vi "nanocal -- nuclear schottky fit -- 2x2 -- V9.vi"() -> ()   [LabVIEW 2021] (continued)
\"στS\" -> 0.003636352111   ,  \"στN\" -> 0.036322417436    |>   , \n\"IDS0184_210310_RAW_cal__sam_\" ->   <|    \"ζ\" -> 0.215697702358   ,  \"τ1\" -> 0.095971807771   ,  \"τS\" -> 0.069319630290   ,  \"τN\" -> 0.366712218878   ,  \"τC\" -> 0.001526252261   ,  \"κ0\" -> 0.000000000784   ,  \"mm1\" -> 0.000266752031   ,  \"mm2\" -> 0.013373263674   ,  \"mm3\" -> 0.613940961515   ,  \"T\" -> 0.148000000000   ,  \"B\" -> 12.000000000000   ,  \"θ\" -> 90.000000000000   ,  \"Reoff\" -> 0.000000000000   ,  \"Imoff\" -> 0.000000000000   ,  \"στ1\" -> 0.000000000000   ,  \"στS\" -> 0.000000000000   ,  \"στN\" -> 0.000000000000    |>   , \n\"IDS0185_210310_RAW_cal__ref_\" ->   <|    \"ζ\" -> 0.175626342721   ,  \"τ1\" -> 0.068013297959   ,  \"τS\" -> 0.031455235747   ,  \"τN\" -> 0.088683010169   ,  \"τC\" -> 0.000955517601   ,  \"κ0\" -> 0.000000001059   ,  \"mm1\" -> 0.000139645447   ,  \"mm2\" -> 0.013049177780   ,  \"mm3\" -> 0.197017679000   ,  \"T\" -> 0.197000000000   ,  \"B\" -> 12.000000000000   ,  \"θ\" -> 90.000000000000   ,  \"Reoff\" -> -34453061.224489793200   ,  \"Imoff\" -> 0.000000000000   ,  \"στ1\" -> 0.004608846817   ,  \"στS\" -> 0.000610901813   ,  \"στN\" -> 0.004550742696    |>   , \n\"IDS0185_210310_RAW_cal__sam_\" ->   <|    \"ζ\" -> 0.139117463690   ,  \"τ1\" -> 0.070330410174   ,  \"τS\" -> 0.040829719954   ,  \"τN\" -> 0.122434321115   ,  \"τC\" -> 0.001436112939   ,  \"κ0\" -> 0.000000001208   ,  \"mm1\" -> 0.000170710071   ,  \"mm2\" -> 0.013785404893   ,  \"mm3\" -> 0.243787328523   ,  \"T\" -> 0.197000000000   ,  \"B\" -> 12.000000000000   ,  \"θ\" -> 90.000000000000   ,  \"Reoff\" -> 0.000000000000   ,  \"Imoff\" -> 0.000000000000   ,  \"στ1\" -> 0.000000000000   ,  \"στS\" -> 0.000000000000   ,  \"στN\" -> 0.000000000000    |>   , \n\"IDS0186_210310_RAW_cal__ref_\" ->   <|    \"ζ\" -> 0.101402144849   ,  \"τ1\" -> 0.051259228694   ,  \"τS\" -> 0.026993470844   ,  \"τN\" -> 0.035386078801   ,  \"τC\" -> 0.001239642629   ,  \"κ0\" -> 0.000000001363   ,  \"mm1\" -> 0.000109940153   ,  \"mm2\" -> 0.014897296966   ,  \"mm3\" -> 0.106196603977   ,  \"T\" -> 0.249000000000   ,  \"B\" -> 12.000000000000   ,  \"θ\" -> 90.000000000000   ,  \"Reoff\" -> -14000000.000000000000   ,  \"Imoff\" -> 0.000000000000   ,  \"στ1\" -> 0.003203070466   ,  \"στS\" -> 0.000314021587   ,  \"στN\" -> 0.001544007051    |>   , \n\"IDS0186_210310_RAW_cal__sam_\" ->   <|    \"ζ\" -> 0.079912790251   ,  \"τ1\" -> 0.053932962768   ,  \"τS\" -> 0.033847624645   ,  \"τN\" -> 0.047947649984   ,  \"τC\" -> 0.001828917906   ,  \"κ0\" -> 0.000000001546   ,  \"mm1\" -> 0.000129305669   ,  \"mm2\" -> 0.016142481427   ,  \"mm3\" -> 0.127821856832   ,  \"T\" -> 0.249000000000   ,  \"B\" -> 12.000000000000   ,  \"θ\" -> 90.000000000000   ,  \"Reoff\" -> 0.000000000000   ,  \"Imoff\" -> 0.000000000000   ,  \"στ1\" -> 0.000000000000   ,  \"στS\" -> 0.000000000000   ,  \"στN\" -> 0.000000000000    |>   , \n\"IDS0187_210310_RAW_cal__ref_\" ->   <|    \"ζ\" -> 0.070400852728   ,  \"τ1\" -> 0.043683571138   ,  \"τS\" -> 0.023747872987   ,  \"τN\" -> 0.017566907569   ,  \"τC\" -> 0.001811397979   ,  \"κ0\" -> 0.000000001742   ,  \"mm1\" -> 0.000111656339   ,  \"mm2\" -> 0.016123687864   ,  \"mm3\" -> 0.073483001252   ,  \"T\" -> 0.300000000000   ,  \"B\" -> 12.000000000000   ,  \"θ\" -> 90.000000000000   ,  \"Reoff\" -> -7469879.518072288490   ,  \"Imoff\" -> 0.000000000000   ,  \"στ1\" -> 0.006425128340   ,  \"στS\" -> 0.000860913040   ,  \"στN\" -> 0.000000000000    |>   , \n\"IDS0187_210310_RAW_cal__sam_\" ->   <|    \"ζ\" -> 0.057938569833   ,  \"τ1\" -> 0.045244527663   ,  \"τS\" -> 0.029709028064   ,  \"τN\" -> 0.023577376257   ,  \"τC\" -> 0.002006607539   ,  \"κ0\" -> 0.000000001948   ,  \"mm1\" -> 0.000103608352   ,  \"mm2\" -> 0.017542867394   ,  \"mm3\" -> 0.085978401835   ,  \"T\" -> 0.300000000000   ,  \"B\" -> 12.000000000000   ,  \"θ\" -> 90.000000000000   ,  \"Reoff\" -> 0.000000000000   ,  \"Imoff\" -> 0.000000000000   ,  \"στ1\" -> 0.000000000000   ,  \"στS\" -> 0.000000000000   ,  \"στN\" -> 0.000000000000    |>   , \n\"IDS0188_210310_RAW_cal__ref_\" ->   <|    \"ζ\" -> 0.052056900695   ,  \"τ1\" -> 0.037832738296   ,  \"τS\" -> 0.021653292165   ,  \"τN\" -> 0.010363134799   ,  \"τC\" -> 0.002302160053   ,  \"κ0\" -> 0.000000002117   ,  \"mm1\" -> 0.000103876216   ,  \"mm2\" -> 0.016526845939   ,  \"mm3\" -> 0.057187279117   ,  \"T\" -> 0.360000000000   ,  \"B\" -> 12.000000000000   ,  \"θ\" -> 90.000000000000   ,  \"Reoff\" -> -4033132.530120491980   ,  \"Imoff\" -> 0.000000000000   ,  \"στ1\" -> 0.008023460591   ,  \"στS\" -> 0.000770743330   ,  \"στN\" -> 0.000000000000    |>   , \n\"IDS0188_210310_RAW_cal__sam_\" ->   <|    \"ζ\" -> 0.044154556051   ,  \"τ1\" -> 0.038823125235   ,  \"τS\" -> 0.027069314930   ,  \"τN\" -> 0.013601990730   ,  \"τC\" -> 0.002287979276   ,  \"κ0\" -> 0.000000002359   ,  \"mm1\" -> 0.000089763345   ,  \"mm2\" -> 0.018083678254   ,  \"mm3\" -> 0.065404792018   ,  \"T\" -> 0.360000000000   ,  \"B\" -> 12.000000000000   ,  \"θ\" -> 90.000000000000   ,  \"Reoff\" -> 0.000000000000   ,  \"Imoff\" -> 0.000000000000   ,  \"στ1\" -> 0.000000000000   ,  \"στS\" -> 0.000000000000   ,  \"στN\" -> 0.000000000000    |>   , \n\"IDS0189_210310_RAW_cal__ref_\" ->   <|    \"ζ\" -> 0.040604780260   ,  \"τ1\" -> 0.030361089686   ,  \"τS\" -> 0.019771781814   ,  \"τN\" -> 0.005325171714   ,  \"τC\" -> 0.002699153711   ,  \"κ0\" -> 0.000000002668   ,  \"mm1\" -> 0.000093474055   ,  \"mm2\" -> 0.016547199805   ,  \"mm3\" -> 0.042535579348   ,  \"T\" -> 0.430000000000   ,  \"B\" -> 12.000000000000   ,  \"θ\" -> 90.000000000000   ,  \"Reoff\" -> -3126506.024096369740   ,  \"Imoff\" -> 0.000000000000   ,  \"στ1\" -> 0.010974863923   ,  \"στS\" -> 0.000726728157   ,  \"στN\" -> 0.000000000000    |>   , \n\"IDS0189_210310_RAW_cal__sam_\" ->   <|    \"ζ\" -> 0.032748569996   ,  \"τ1\" -> 0.031072007290   ,  \"τS\" -> 0.024343937548   ,  \"τN\" -> 0.006961654481   ,  \"τC\" -> 0.002967111565   ,  \"κ0\" -> 0.000000002964   ,  \"mm1\" -> 0.000084402249   ,  \"mm2\" -> 0.018055855929   ,  \"mm3\" -> 0.048229666078   ,  \"T\" -> 0.430000000000   ,  \"B\" -> 12.000000000000   ,  \"θ\" -> 90.000000000000   ,  \"Reoff\" -> 0.000000000000   ,  \"Imoff\" -> 0.000000000000   ,  \"στ1\" -> 0.000000000000   ,  \"στS\" -> 0.000000000000   ,  \"στN\" -> 0.000000000000    |>   , \n\"IDS0190_210310_RAW_cal__ref_\" ->   <|    \"ζ\" -> 0.030700897923   ,  \"τ1\" -> 0.026935085078   ,  \"τS\" -> 0.018364864329   ,  \"τN\" -> 0.002898516959   ,  \"τC\" -> 0.003150649099   ,  \"κ0\" -> 0.000000003342   ,  \"mm1\" -> 0.000080744936   ,  \"mm2\" -> 0.016939553323   ,  \"mm3\" -> 0.034981622105   ,  \"T\" -> 0.512000000000   ,  \"B\" -> 12.000000000000   ,  \"θ\" -> 90.000000000000   ,  \"Reoff\" -> 0.000000000000   ,  \"Imoff\" -> 0.000000000000   ,  \"στ1\" -> 0.000000000000   ,  \"στS\" -> 0.000000000000   ,  \"στN\" -> 0.000000000000    |>   , \n\"IDS0190_210310_RAW_cal__sam_\" ->   <|    \"ζ\" -> 0.027599263457   ,  \"τ1\" -> 0.026239105728   ,  \"τS\" -> 0.022370859308   ,  \"τN\" -> 0.003857632966   ,  \"τC\" -> 0.003499360499   ,  \"κ0\" -> 0.000000003681   ,  \"mm1\" -> 0.000081816106   ,  \"mm2\" -> 0.017901054668   ,  \"mm3\" -> 0.038707974796   ,  \"T\" -> 0.512000000000   ,  \"B\" -> 12.000000000000   ,  \"θ\" -> 90.000000000000   ,  \"Reoff\" -> 0.000000000000   ,  \"Imoff\" -> 0.000000000000   ,  \"στ1\" -> 0.000000000000   ,  \"στS\" -> 0.000000000000   ,  \"στN\" -> 0.000000000000    |>   , \n\"IDS0191_210310_RAW_cal__ref_\" ->   <|    \"ζ\" -> 0.025322625458   ,  \"τ1\" -> 0.023401812401   ,  \"τS\" -> 0.017347416709   ,  \"τN\" -> 0.002020498851   ,  \"τC\" -> 0.003594259467   ,  \"κ0\" -> 0.000000003970   ,  \"mm1\" -> 0.000074098080   ,  \"mm2\" -> 0.016429541452   ,  \"mm3\" -> 0.030350794367   ,  \"T\" -> 0.610000000000   ,  \"B\" -> 12.000000000000   ,  \"θ\" -> 90.000000000000   ,  \"Reoff\" -> 0.000000000000   ,  \"Imoff\" -> 0.000000000000   ,  \"στ1\" -> 0.000000000000   ,  \"στS\" -> 0.000000000000   ,  \"στN\" -> 0.000000000000    |>   , \n\"IDS0191_210310_RAW_cal__sam_\" ->   <|    \"ζ\" -> 0.020568815513   ,  \"τ1\" -> 0.023045965648   ,  \"τS\" -> 0.020791387386   ,  \"τN\" -> 0.002229171297   ,  \"τC\" -> 0.004427475438   ,  \"κ0\" -> 0.000000004398   ,  \"mm1\" -> 0.000074037290   ,  \"mm2\" -> 0.017820522459   ,  \"mm3\" -> 0.033072945644   ,  \"T\" -> 0.610000000000   ,  \"B\" -> 12.000000000000   ,  \"θ\" -> 90.000000000000   ,  \"Reoff\" -> 0.000000000000   ,  \"Imoff\" -> 0.000000000000   ,  \"στ1\" -> 0.000000000000   ,  \"στS\" -> 0.000000000000   ,  \"στN\" -> 0.000000000000    |>   , \n\"IDS0192_210310_RAW_cal__ref_\" ->   <|    \"ζ\" -> 0.022100596026   ,  \"τ1\" -> 0.020519097823   ,  \"τS\" -> 0.015555141042   ,  \"τN\" -> 0.000889956832   ,  \"τC\" -> 0.004354791503   ,  \"κ0\" -> 0.000000005560   ,  \"mm1\" -> 0.000074184851   ,  \"mm2\" -> 0.016476573734   ,  \"mm3\" -> 0.025131675080   ,  \"T\" -> 0.810000000000   ,  \"B\" -> 12.000000000000   ,  \"θ\" -> 90.000000000000   ,  \"Reoff\" -> 0.000000000000   ,  \"Imoff\" -> 0.000000000000   ,  \"στ1\" -> 0.000000000000   ,  \"στS\" -> 0.000000000000   ,  \"στN\" -> 0.000000000000    |>   , \n\"IDS0192_210310_RAW_cal__sam_\" ->   <|    \"ζ\" -> 0.016548170999   ,  \"τ1\" -> 0.020108887890   ,  \"τS\" -> 0.018558394948   ,  \"τN\" -> 0.001160732495   ,  \"τC\" -> 0.004746126241   ,  \"κ0\" -> 0.000000005882   ,  \"mm1\" -> 0.000061890920   ,  \"mm2\" -> 0.017029753868   ,  \"mm3\" -> 0.027808812278   ,  \"T\" -> 0.810000000000   ,  \"B\" -> 12.000000000000   ,  \"θ\" -> 90.000000000000   ,  \"Reoff\" -> 0.000000000000   ,  \"Imoff\" -> 0.000000000000   ,  \"στ1\" -> 0.000000000000   ,  \"στS\" -> 0.000000000000   ,  \"στN\" -> 0.000000000000    |>   , \n\"IDS0193_210310_RAW_cal__ref_\" ->   <|    \"ζ\" -> 0.019733832284   ,  \"τ1\" -> 0.020049224921   ,  \"τS\" -> 0.014230397771   ,  \"τN\" -> 0.000441389176   ,  \"τC\" -> 0.004438301040   ,  \"κ0\" -> 0.000000007769   ,  \"mm1\" -> 0.000066001229   ,  \"mm2\" -> 0.016667650670   ,  \"mm3\" -> 0.022715191592   ,  \"T\" -> 1.100000000000   ,  \"B\" -> 12.000000000000   ,  \"θ\" -> 90.000000000000   ,  \"Reoff\" -> -579591.836734693729   ,  \"Imoff\" -> 0.000000000000   ,  \"στ1\" -> 0.001958401015   ,  \"στS\" -> 0.000185837880   ,  \"στN\" -> 0.000023607479    |>   , \n\"IDS0193_210310_RAW_cal__sam_\" ->   <|    \"ζ\" -> 0.014495870556   ,  \"τ1\" -> 0.019990087457   ,  \"τS\" -> 0.016832201384   ,  \"τN\" -> 0.000455517238   ,  \"τC\" -> 0.005555782498   ,  \"κ0\" -> 0.000000008420   ,  \"mm1\" -> 0.000060055560   ,  \"mm2\" -> 0.018114231010   ,  \"mm3\" -> 0.024909902538   ,  \"T\" -> 1.100000000000   ,  \"B\" -> 12.000000000000   ,  \"θ\" -> 90.000000000000   ,  \"Reoff\" -> 0.000000000000   ,  \"Imoff\" -> 0.000000000000   ,  \"στ1\" -> 0.000000000000   ,  \"στS\" -> 0.000000000000   ,  \"στN\" -> 0.000000000000    |>   , \n\"IDS0194_210310_RAW_cal__ref_\" ->   <|    \"ζ\" -> 0.017005565439   ,  \"τ1\" -> 0.018296939194   ,  \"τS\" -> 0.010720873838   ,  \"τN\" -> 0.000107866268   ,  \"τC\" -> 0.005258546332   ,  \"κ0\" -> 0.000000013438   ,  \"mm1\" -> 0.000059538412   ,  \"mm2\" -> 0.015496319396   ,  \"mm3\" -> 0.019012516672   ,  \"T\" -> 1.800000000000   ,  \"B\" -> 12.000000000000   ,  \"θ\" -> 90.000000000000   ,  \"Reoff\" -> -212244.897959183668   ,  \"Imoff\" -> 0.000000000000   ,  \"στ1\" -> 0.002365395805   ,  \"στS\" -> 0.000151267188   ,  \"στN\" -> 0.000004998661    |>   , \n\"IDS0194_210310_RAW_cal__sam_\" ->   <|    \"ζ\" -> 0.014043763709   ,  \"τ1\" -> 0.018292068543   ,  \"τS\" -> 0.011311396743   ,  \"τN\" -> 0.000128802259   ,  \"τC\" -> 0.008087849636   ,  \"κ0\" -> 0.000000014258   ,  \"mm1\" -> 0.000065912054   ,  \"mm2\" -> 0.017276417784   ,  \"mm3\" -> 0.020638450794   ,  \"T\" -> 1.800000000000   ,  \"B\" -> 12.000000000000   ,  \"θ\" -> 90.000000000000   ,  \"Reoff\" -> 0.000000000000   ,  \"Imoff\" -> 0.000000000000   ,  \"στ1\" -> 0.000000000000   ,  \"στS\" -> 0.000000000000   ,  \"στN\" -> 0.000000000000    |>   , \n\"IDS0195_210310_RAW_cal__ref_\" ->   <|    \"ζ\" -> 0.019004360175   ,  \"τ1\" -> 0.018297498699   ,  \"τS\" -> 0.007362425348   ,  \"τN\" -> 0.000028493035   ,  \"τC\" -> 0.005091066429   ,  \"κ0\" -> 0.000000023928   ,  \"mm1\" -> 0.000056820022   ,  \"mm2\" -> 0.012474579286   ,  \"mm3\" -> 0.018388543878   ,  \"T\" -> 3.000000000000   ,  \"B\" -> 12.000000000000   ,  \"θ\" -> 90.000000000000   ,  \"Reoff\" -> -126530.612244897755   ,  \"Imoff\" -> 0.000000000000   ,  \"στ1\" -> 0.002124476662   ,  \"στS\" -> 0.000135263325   ,  \"στN\" -> 0.000001554239    |>   , \n\"IDS0195_210310_RAW_cal__sam_\" ->   <|    \"ζ\" -> 0.016187684631   ,  \"τ1\" -> 0.018325345271   ,  \"τS\" -> 0.007510087776   ,  \"τN\" -> 0.000028419157   ,  \"τC\" -> 0.008115463080   ,  \"κ0\" -> 0.000000024747   ,  \"mm1\" -> 0.000062903858   ,  \"mm2\" -> 0.015524812312   ,  \"mm3\" -> 0.018513630087   ,  \"T\" -> 3.000000000000   ,  \"B\" -> 12.000000000000   ,  \"θ\" -> 90.000000000000   ,  \"Reoff\" -> 0.000000000000   ,  \"Imoff\" -> 0.000000000000   ,  \"στ1\" -> 0.000000000000   ,  \"στS\" -> 0.000000000000   ,  \"στN\" -> 0.000000000000    |>   , \n\"IDS0196_210310_RAW_cal__ref_\" ->   <|    \"ζ\" -> 0.019836117240   ,  \"τ1\" -> 0.012821319030   ,  \"τS\" -> 0.004629754482   ,  \"τN\" -> 0.000007000803   ,  \"τC\" -> 0.003894449698   ,  \"κ0\" -> 0.000000058909   ,  \"mm1\" -> 0.000041711868   ,  \"mm2\" -> 0.008560043716   ,  \"mm3\" -> 0.012842743651   ,  \"T\" -> 5.700000000000   ,  \"B\" -> 12.000000000000   ,  \"θ\" -> 90.000000000000   ,  \"Reoff\" -> -53061.224489795742   ,  \"Imoff\" -> 0.000000000000   ,  \"στ1\" -> 0.001499698483   ,  \"στS\" -> 0.000975702088   ,  \"στN\" -> 0.000003238614    |>   , \n\"IDS0196_210310_RAW_cal__sam_\" ->   <|    \"ζ\" -> 0.027897403691   ,  \"τ1\" -> 0.014639690770   ,  \"τS\" -> 0.004105291179   ,  \"τN\" -> 0.000006999171   ,  \"τC\" -> 0.007414449545   ,  \"κ0\" -> 0.000000059701   ,  \"mm1\" -> 0.000073450671   ,  \"mm2\" -> 0.011534391407   ,  \"mm3\" -> 0.014673310811   ,  \"T\" -> 5.700000000000   ,  \"B\" -> 12.000000000000   ,  \"θ\" -> 90.000000000000   ,  \"Reoff\" -> 0.000000000000   ,  \"Imoff\" -> 0.000000000000   ,  \"στ1\" -> 0.000000000000   ,  \"στS\" -> 0.000000000000   ,  \"στN\" -> 0.000000000000    |>   , \n\"IDS0208_210310_RAW_cal__ref_\" ->   <|    \"ζ\" -> 0.000000000000   ,  \"τ1\" -> 0.000000000000   ,  \"τS\" -> 0.000000000000   ,  \"τN\" -> 0.000000000000   ,  \"τC\" -> 0.000000000000   ,  \"κ0\" -> 0.000000000000   ,  \"mm1\" -> 0.000000000000   ,  \"mm2\" -> 0.000000000000   ,  \"mm3\" -> 0.000000000000   ,  \"T\" -> 0.197000000000   ,  \"B\" -> 0.000000000000   ,  \"θ\" -> 0.000000000000   ,  \"Reoff\" -> 0.000000000000   ,  \"Imoff\" -> 0.000000000000   ,  \"στ1\" -> 0.000000000000   ,  \"στS\" -> 0.000000000000   ,  \"στN\" -> 0.000000000000    |>   , \n\"IDS0208_210310_RAW_cal__sam_\" ->   <|    \"ζ\" -> 0.000000000000   ,  \"τ1\" -> 0.000000000000   ,  \"τS\" -> 0.000000000000   ,  \"τN\" -> 0.000000000000   ,  \"τC\" -> 0.000000000000   ,  \"κ0\" -> 0.000000000000   ,  \"mm1\" -> 0.000000000000   ,  \"mm2\" -> 0.000000000000   ,  \"mm3\" -> 0.000000000000   ,  \"T\" -> 0.197000000000   ,  \"B\" -> 0.000000000000   ,  \"θ\" -> 0.000000000000   ,  \"Reoff\" -> 0.000000000000   ,  \"Imoff\" -> 0.000000000000   ,  \"στ1\" -> 0.000000000000   ,  \"στS\" -> 0.000000000000   ,  \"στN\" -> 0.000000000000    |>   , \n\"IDS0209_210310_RAW_cal__ref_\" ->   <|    \"ζ\" -> 0.163571654798   ,  \"τ1\" -> 0.020520714675   ,  \"τS\" -> 0.073117323271   ,  \"τN\" -> 0.020627224399   ,  \"τC\" -> 0.001336341391   ,  \"κ0\" -> 0.000000001061   ,  \"mm1\" -> 0.000185345173   ,  \"mm2\" -> 0.015331340913   ,  \"mm3\" -> 0.115418868440   ,  \"T\" -> 0.197000000000   ,  \"B\" -> 0.000000000000   ,  \"θ\" -> 0.000000000000   ,  \"Reoff\" -> 0.000000000000   ,  \"Imoff\" -> 0.000000000000   ,  \"στ1\" -> 0.000000000000   ,  \"στS\" -> 0.000000000000   ,  \"στN\" -> 0.000000000000    |>   , \n\"IDS0209_210310_RAW_cal__sam_\" ->   <|    \"ζ\" -> 0.132901556203   ,  \"τ1\" -> 0.022795175616   ,  \"τS\" -> 0.082481385864   ,  \"τN\" -> 0.041432545456   ,  \"τC\" -> 0.001408424074   ,  \"κ0\" -> 0.000000001182   ,  \"mm1\" -> 0.000163042447   ,  \"mm2\" -> 0.014386869823   ,  \"mm3\" -> 0.150035973048   ,  \"T\" -> 0.197000000000   ,  \"B\" -> 0.000000000000   ,  \"θ\" -> 0.000000000000   ,  \"Reoff\" -> 0.000000000000   ,  \"Imoff\" -> 0.000000000000   ,  \"στ1\" -> 0.000000000000   ,  \"στS\" -> 0.000000000000   ,  \"στN\" -> 0.000000000000    |>   , \n\"IDS0210_210310_RAW_cal__ref_\" ->   <|    \"ζ\" -> 0.000000000000   ,  \"τ1\" -> 0.000000000000   ,  \"τS\" -> 0.000000000000   ,  \"τN\" -> 0.000000000000   ,  \"τC\" -> 0.000000000000   ,  \"κ0\" -> 0.000000000000   ,  \"mm1\" -> 0.000000000000   ,  \"mm2\" -> 0.000000000000   ,  \"mm3\" -> 0.000000000000   ,  \"T\" -> 0.148000000000   ,  \"B\" -> 6.000000000000   ,  \"θ\" -> 0.000000000000   ,  \"Reoff\" -> 0.000000000000   ,  \"Imoff\" -> 0.000000000000   ,  \"στ1\" -> 0.000000000000   ,  \"στS\" -> 0.000000000000   ,  \"στN\" -> 0.000000000000    |>   , \n\"IDS0210_210310_RAW_cal__sam_\" ->   <|    \"ζ\" -> 0.000000000000   ,  \"τ1\" -> 0.000000000000   ,  \"τS\" -> 0.000000000000   ,  \"τN\" -> 0.000000000000   ,  \"τC\" -> 0.000000000000   ,  \"κ0\" -> 0.000000000000   ,  \"mm1\" -> 0.000000000000   ,  \"mm2\" -> 0.000000000000   ,  \"mm3\" -> 0.000000000000   ,  \"T\" -> 0.148000000000   ,  \"B\" -> 6.000000000000   ,  \"θ\" -> 0.000000000000   ,  \"Reoff\" -> 0.000000000000   ,  \"Imoff\" -> 0.000000000000   ,  \"στ1\" -> 0.000000000000   ,  \"στS\" -> 0.000000000000   ,  \"στN\" -> 0.000000000000    |>   , \n\"IDS0211_210310_RAW_cal__ref_\" ->   <|    \"ζ\" -> 0.160882265826   ,  \"τ1\" -> 0.034919932965   ,  \"τS\" -> 0.043973777096   ,  \"τN\" -> 0.047289018614   ,  \"τC\" -> 0.001339652100   ,  \"κ0\" -> 0.000000001069   ,  \"mm1\" -> 0.000181515969   ,  \"mm2\" -> 0.014272071349   ,  \"mm3\" -> 0.127751358817   ,  \"T\" -> 0.197000000000   ,  \"B\" -> 9.000000000000   ,  \"θ\" -> 0.000000000000   ,  \"Reoff\" -> 0.000000000000   ,  \"Imoff\" -> 0.000000000000   ,  \"στ1\" -> 0.000000000000   ,  \"στS\" -> 0.000000000000   ,  \"στN\" -> 0.000000000000    |>   , \n\"IDS0211_210310_RAW_cal__sam_\" ->   <|    \"ζ\" -> 0.132534999612   ,  \"τ1\" -> 0.042581417401   ,  \"τS\" -> 0.054103824371   ,  \"τN\" -> 0.072163013930   ,  \"τC\" -> 0.001421040158   ,  \"κ0\" -> 0.000000001190   ,  \"mm1\" -> 0.000162934689   ,  \"mm2\" -> 0.015546305497   ,  \"mm3\" -> 0.171294831040   ,  \"T\" -> 0.197000000000   ,  \"B\" -> 9.000000000000   ,  \"θ\" -> 0.000000000000   ,  \"Reoff\" -> 0.000000000000   ,  \"Imoff\" -> 0.000000000000   ,  \"στ1\" -> 0.000000000000   ,  \"στS\" -> 0.000000000000   ,  \"στN\" -> 0.000000000000    |>   , \n\"IDS0212_210310_RAW_cal__ref_\" ->   <|    \"ζ\" -> 0.154351103049   ,  \"τ1\" -> 0.051844552801   ,  \"τS\" -> 0.034651211615   ,  \"τN\" -> 0.065884588100   ,  \"τC\" -> 0.001166375427   ,  \"κ0\" -> 0.000000001084   ,  \"mm1\" -> 0.000152080810   ,  \"mm2\" -> 0.013701664106   ,  \"mm3\" -> 0.155210794609   ,  \"T\" -> 0.197000000000   ,  \"B\" -> 11.000000000000   ,  \"θ\" -> 0.000000000000   ,  \"Reoff\" -> 0.000000000000   ,  \"Imoff\" -> 0.000000000000   ,  \"στ1\" -> 0.000000000000   ,  \"στS\" -> 0.000000000000   ,  \"στN\" -> 0.000000000000    |>   , \n\"IDS0212_210310_RAW_cal__sam_\" ->   <|    \"ζ\" -> 0.124414912597   ,  \"τ1\" -> 0.052685716706   ,  \"τS\" -> 0.041788480794   ,  \"τN\" -> 0.092820346766   ,  \"τC\" -> 0.001183564004   ,  \"κ0\" -> 0.000000001217   ,  \"mm1\" -> 0.000128067207   ,  \"mm2\" -> 0.013191279693   ,  \"mm3\" -> 0.191906106886   ,  \"T\" -> 0.197000000000   ,  \"B\" -> 11.000000000000   ,  \"θ\" -> 0.000000000000   ,  \"Reoff\" -> 0.000000000000   ,  \"Imoff\" -> 0.000000000000   ,  \"στ1\" -> 0.000000000000   ,  \"στS\" -> 0.000000000000   ,  \"στN\" -> 0.000000000000    |>   , \n\"IDS0213_210310_RAW_cal__ref_\" ->   <|    \"ζ\" -> 0.158514180755   ,  \"τ1\" -> 0.046388884826   ,  \"τS\" -> 0.038847986012   ,  \"τN\" -> 0.058494864948   ,  \"τC\" -> 0.001325817289   ,  \"κ0\" -> 0.000000001072   ,  \"mm1\" -> 0.000176864175   ,  \"mm2\" -> 0.014706895751   ,  \"mm3\" -> 0.145604015421   ,  \"T\" -> 0.197000000000   ,  \"B\" -> 10.000000000000   ,  \"θ\" -> 0.000000000000   ,  \"Reoff\" -> 0.000000000000   ,  \"Imoff\" -> 0.000000000000   ,  \"στ1\" -> 0.000000000000   ,  \"στS\" -> 0.000000000000   ,  \"στN\" -> 0.000000000000    |>   , \n\"IDS0213_210310_RAW_cal__sam_\" ->   <|    \"ζ\" -> 0.130083148284   ,  \"τ1\" -> 0.046211117525   ,  \"τS\" -> 0.046173592526   ,  \"τN\" -> 0.081942172735   ,  \"τC\" -> 0.001380184863   ,  \"κ0\" -> 0.000000001209   ,  \"mm1\" -> 0.000155206642   ,  \"mm2\" -> 0.013836953800   ,  \"mm3\" -> 0.178380609297   ,  \"T\" -> 0.197000000000   ,  \"B\" -> 10.000000000000   ,  \"θ\" -> 0.000000000000   ,  \"Reoff\" -> 0.000000000000   ,  \"Imoff\" -> 0.000000000000   ,  \"στ1\" -> 0.000000000000   ,  \"στS\" -> 0.000000000000   ,  \"στN\" -> 0.000000000000    |>   , \n\"IDS0214_210310_RAW_cal__ref_\" ->   <|    \"ζ\" -> 0.154362032240   ,  \"τ1\" -> 0.030258273194   ,  \"τS\" -> 0.049523350330   ,  \"τN\" -> 0.040015703513   ,  \"τC\" -> 0.001328953616   ,  \"κ0\" -> 0.000000001075   ,  \"mm1\" -> 0.000174173720   ,  \"mm2\" -> 0.014698349376   ,  \"mm3\" -> 0.120075187874   ,  \"T\" -> 0.197000000000   ,  \"B\" -> 8.000000000000   ,  \"θ\" -> 0.000000000000   ,  \"Reoff\" -> 0.000000000000   ,  \"Imoff\" -> 0.000000000000   ,  \"στ1\" -> 0.000000000000   ,  \"στS\" -> 0.000000000000   ,  \"στN\" -> 0.000000000000    |>   , \n\"IDS0214_210310_RAW_cal__sam_\" ->   <|    \"ζ\" -> 0.126440702434   ,  \"τ1\" -> 0.034118036572   ,  \"τS\" -> 0.060921114440   ,  \"τN\" -> 0.059832148427   ,  \"τC\" -> 0.001404471084   ,  \"κ0\" -> 0.000000001199   ,  \"mm1\" -> 0.000154817132   ,  \"mm2\" -> 0.015271462818   ,  \"mm3\" -> 0.156117617951   ,  \"T\" -> 0.197000000000   ,  \"B\" -> 8.000000000000   ,  \"θ\" -> 0.000000000000   ,  \"Reoff\" -> 0.000000000000   ,  \"Imoff\" -> 0.000000000000   ,  \"στ1\" -> 0.000000000000   ,  \"στS\" -> 0.000000000000   ,  \"στN\" -> 0.000000000000    |>   , \n\"IDS0215_210310_RAW_cal__ref_\" ->   <|    \"ζ\" -> 0.162645417184   ,  \"τ1\" -> 0.023693851446   ,  \"τS\" -> 0.062400062170   ,  \"τN\" -> 0.026326088223   ,  \"τC\" -> 0.001322053294   ,  \"κ0\" -> 0.000000001070   ,  \"mm1\" -> 0.000182075033   ,  \"mm2\" -> 0.015525359924   ,  \"mm3\" -> 0.112465521923   ,  \"T\" -> 0.197000000000   ,  \"B\" -> 7.000000000000   ,  \"θ\" -> 0.000000000000   ,  \"Reoff\" -> 0.000000000000   ,  \"Imoff\" -> 0.000000000000   ,  \"στ1\" -> 0.000000000000   ,  \"στS\" -> 0.000000000000   ,  \"στN\" -> 0.000000000000    |>   , \n\"IDS0215_210310_RAW_cal__sam_\" ->   <|    \"ζ\" -> 0.131383255045   ,  \"τ1\" -> 0.026827335842   ,  \"τS\" -> 0.071725959535   ,  \"τN\" -> 0.047510049318   ,  \"τC\" -> 0.001407613780   ,  \"κ0\" -> 0.000000001187   ,  \"mm1\" -> 0.000160977956   ,  \"mm2\" -> 0.014932130994   ,  \"mm3\" -> 0.148043464486   ,  \"T\" -> 0.197000000000   ,  \"B\" -> 7.000000000000   ,  \"θ\" -> 0.000000000000   ,  \"Reoff\" -> 0.000000000000   ,  \"Imoff\" -> 0.000000000000   ,  \"στ1\" -> 0.000000000000   ,  \"στS\" -> 0.000000000000   ,  \"στN\" -> 0.000000000000    |>   , \n\"IDS0216_210310_RAW_cal__ref_\" ->   <|    \"ζ\" -> 0.149904026692   ,  \"τ1\" -> 0.020347243982   ,  \"τS\" -> 0.075273674904   ,  \"τN\" -> 0.020640082408   ,  \"τC\" -> 0.001432916876   ,  \"κ0\" -> 0.000000001050   ,  \"mm1\" -> 0.000184134986   ,  \"mm2\" -> 0.015328528282   ,  \"mm3\" -> 0.116559113338   ,  \"T\" -> 0.197000000000   ,  \"B\" -> 5.000000000000   ,  \"θ\" -> 0.000000000000   ,  \"Reoff\" -> 0.000000000000   ,  \"Imoff\" -> 0.000000000000   ,  \"στ1\" -> 0.000000000000   ,  \"στS\" -> 0.000000000000   ,  \"στN\" -> 0.000000000000    |>   , \n\"IDS0216_210310_RAW_cal__sam_\" ->   <|    \"ζ\" -> 0.125455081262   ,  \"τ1\" -> 0.021777951907   ,  \"τS\" -> 0.089086097551   ,  \"τN\" -> 0.033580911935   ,  \"τC\" -> 0.001437991682   ,  \"κ0\" -> 0.000000001167   ,  \"mm1\" -> 0.000158268021   ,  \"mm2\" -> 0.015150793318   ,  \"mm3\" -> 0.145963091379   ,  \"T\" -> 0.197000000000   ,  \"B\" -> 5.000000000000   ,  \"θ\" -> 0.000000000000   ,  \"Reoff\" -> 0.000000000000   ,  \"Imoff\" -> 0.000000000000   ,  \"στ1\" -> 0.000000000000   ,  \"στS\" -> 0.000000000000   ,  \"στN\" -> 0.000000000000    |>   , \n\"IDS0217_210310_RAW_cal__ref_\" ->   <|    \"ζ\" -> 0.121305227705   ,  \"τ1\" -> 0.032098202143   ,  \"τS\" -> 0.011865067519   ,  \"τN\" -> 0.005878702730   ,  \"τC\" -> 0.002147559783   ,  \"κ0\" -> 0.000000001032   ,  \"mm1\" -> 0.000202614262   ,  \"mm2\" -> 0.011552455211   ,  \"mm3\" -> 0.042386874792   ,  \"T\" -> 0.197000000000   ,  \"B\" -> 0.000000000000   ,  \"θ\" -> 0.000000000000   ,  \"Reoff\" -> 0.000000000000   ,  \"Imoff\" -> 0.000000000000   ,  \"στ1\" -> 0.000000000000   ,  \"στS\" -> 0.000000000000   ,  \"στN\" -> 0.000000000000    |>   , \n\"IDS0217_210310_RAW_cal__sam_\" ->   <|    \"ζ\" -> 0.101804363109   ,  \"τ1\" -> 0.031947692776   ,  \"τS\" -> 0.014125667853   ,  \"τN\" -> 0.006009042128   ,  \"τC\" -> 0.002323789932   ,  \"κ0\" -> 0.000000001168   ,  \"mm1\" -> 0.000188754224   ,  \"mm2\" -> 0.013103876414   ,  \"mm3\" -> 0.043163363377   ,  \"T\" -> 0.197000000000   ,  \"B\" -> 0.000000000000   ,  \"θ\" -> 0.000000000000   ,  \"Reoff\" -> 0.000000000000   ,  \"Imoff\" -> 0.000000000000   ,  \"στ1\" -> 0.000000000000   ,  \"στS\" -> 0.000000000000   ,  \"στN\" -> 0.000000000000    |>   , \n\"IDS0218_210310_RAW_cal__ref_\" ->   <|    \"ζ\" -> 0.000000000000   ,  \"τ1\" -> 0.000000000000   ,  \"τS\" -> 0.000000000000   ,  \"τN\" -> 0.000000000000   ,  \"τC\" -> 0.000000000000   ,  \"κ0\" -> 0.000000000000   ,  \"mm1\" -> 0.000000000000   ,  \"mm2\" -> 0.000000000000   ,  \"mm3\" -> 0.000000000000   ,  \"T\" -> 1.550000000000   ,  \"B\" -> 0.000000000000   ,  \"θ\" -> 0.000000000000   ,  \"Reoff\" -> 0.000000000000   ,  \"Imoff\" -> 0.000000000000   ,  \"στ1\" -> 0.000000000000   ,  \"στS\" -> 0.000000000000   ,  \"στN\" -> 0.000000000000    |>   , \n\"IDS0218_210310_RAW_cal__sam_\" ->   <|    \"ζ\" -> 0.008537038929   ,  \"τ1\" -> 0.006154643814   ,  \"τS\" -> 0.040521205127   ,  \"τN\" -> 0.000711776675   ,  \"τC\" -> 0.001925410383   ,  \"κ0\" -> 0.000000011800   ,  \"mm1\" -> 0.000015570479   ,  \"mm2\" -> 0.006036709260   ,  \"mm3\" -> 0.043612763831   ,  \"T\" -> 1.550000000000   ,  \"B\" -> 0.000000000000   ,  \"θ\" -> 0.000000000000   ,  \"Reoff\" -> -420408.163265306153   ,  \"Imoff\" -> 0.000000000000   ,  \"στ1\" -> 0.000216261088   ,  \"στS\" -> 0.000541561495   ,  \"στN\" -> 0.000022390164    |>   , \n\"IDS0219_210310_RAW_cal__ref_\" ->   <|    \"ζ\" -> 0.000000000000   ,  \"τ1\" -> 0.000000000000   ,  \"τS\" -> 0.000000000000   ,  \"τN\" -> 0.000000000000   ,  \"τC\" -> 0.000000000000   ,  \"κ0\" -> 0.000000000000   ,  \"mm1\" -> 0.000000000000   ,  \"mm2\" -> 0.000000000000   ,  \"mm3\" -> 0.000000000000   ,  \"T\" -> 1.000000000000   ,  \"B\" -> 0.000000000000   ,  \"θ\" -> 0.000000000000   ,  \"Reoff\" -> 0.000000000000   ,  \"Imoff\" -> 0.000000000000   ,  \"στ1\" -> 0.000000000000   ,  \"στS\" -> 0.000000000000   ,  \"στN\" -> 0.000000000000    |>   , \n\"IDS0219_210310_RAW_cal__sam_\" ->   <|    \"ζ\" -> 0.000000000000   ,  \"τ1\" -> 0.000000000000   ,  \"τS\" -> 0.000000000000   ,  \"τN\" -> 0.000000000000   ,  \"τC\" -> 0.000000000000   ,  \"κ0\" -> 0.000000000000   ,  \"mm1\" -> 0.000000000000   ,  \"mm2\" -> 0.000000000000   ,  \"mm3\" -> 0.000000000000   ,  \"T\" -> 1.000000000000   ,  \"B\" -> 0.000000000000   ,  \"θ\" -> 0.000000000000   ,  \"Reoff\" -> 0.000000000000   ,  \"Imoff\" -> 0.000000000000   ,  \"στ1\" -> 0.000000000000   ,  \"στS\" -> 0.000000000000   ,  \"στN\" -> 0.000000000000    |>   , \n\"IDS0220_210310_RAW_cal__ref_\" ->   <|    \"ζ\" -> 0.000000000000   ,  \"τ1\" -> 0.000000000000   ,  \"τS\" -> 0.000000000000   ,  \"τN\" -> 0.000000000000   ,  \"τC\" -> 0.000000000000   ,  \"κ0\" -> 0.000000000000   ,  \"mm1\" -> 0.000000000000   ,  \"mm2\" -> 0.000000000000   ,  \"mm3\" -> 0.000000000000   ,  \"T\" -> 0.677000000000   ,  \"B\" -> 0.000000000000   ,  \"θ\" -> 0.000000000000   ,  \"Reoff\" -> 0.000000000000   ,  \"Imoff\" -> 0.000000000000   ,  \"στ1\" -> 0.000000000000   ,  \"στS\" -> 0.000000000000   ,  \"στN\" -> 0.000000000000    |>   , \n\"IDS0220_210310_RAW_cal__sam_\" ->   <|    \"ζ\" -> 0.000000000000   ,  \"τ1\" -> 0.000000000000   ,  \"τS\" -> 0.000000000000   ,  \"τN\" -> 0.000000000000   ,  \"τC\" -> 0.000000000000   ,  \"κ0\" -> 0.000000000000   ,  \"mm1\" -> 0.000000000000   ,  \"mm2\" -> 0.000000000000   ,  \"mm3\" -> 0.000000000000   ,  \"T\" -> 0.677000000000   ,  \"B\" -> 0.000000000000   ,  \"θ\" -> 0.000000000000   ,  \"Reoff\" -> 0.000000000000   ,  \"Imoff\" -> 0.000000000000   ,  \"στ1\" -> 0.000000000000   ,  \"στS\" -> 0.000000000000   ,  \"στN\" -> 0.000000000000    |>   , \n\"IDS0224_210310_RAW_cal__ref_\" ->   <|    \"ζ\" -> 0.000000000000   ,  \"τ1\" -> 0.000000000000   ,  \"τS\" -> 0.000000000000   ,  \"τN\" -> 0.000000000000   ,  \"τC\" -> 0.000000000000   ,  \"κ0\" -> 0.000000000000   ,  \"mm1\" -> 0.000000000000   ,  \"mm2\" -> 0.000000000000   ,  \"mm3\" -> 0.000000000000   ,  \"T\" -> 0.000000000000   ,  \"B\" -> 0.000000000000   ,  \"θ\" -> 0.000000000000   ,  \"Reoff\" -> 0.000000000000   ,  \"Imoff\" -> 0.000000000000   ,  \"στ1\" -> 0.000000000000   ,  \"στS\" -> 0.000000000000   ,  \"στN\" -> 0.000000000000    |>   , \n\"IDS0224_210310_RAW_cal__sam_\" ->   <|    \"ζ\" -> 0.000000000000   ,  \"τ1\" -> 0.000000000000   ,  \"τS\" -> 0.000000000000   ,  \"τN\" -> 0.000000000000   ,  \"τC\" -> 0.000000000000   ,  \"κ0\" -> 0.000000000000   ,  \"mm1\" -> 0.000000000000   ,  \"mm2\" -> 0.000000000000   ,  \"mm3\" -> 0.000000000000   ,  \"T\" -> 0.000000000000   ,  \"B\" -> 0.000000000000   ,  \"θ\" -> 0.000000000000   ,  \"Reoff\" -> 0.000000000000   ,  \"Imoff\" -> 0.000000000000   ,  \"στ1\" -> 0.000000000000   ,  \"στS\" -> 0.000000000000   ,  \"στN\" -> 0.000000000000    |>   , \n\"IDS0293_210427_RAW_cal__ref_\" ->   <|    \"ζ\" -> 0.016384838586   ,  \"τ1\" -> 0.013784349529   ,  \"τS\" -> 0.011495286759   ,  \"τN\" -> 0.000117117954   ,  \"τC\" -> 0.004048153799   ,  \"κ0\" -> 0.000000013122   ,  \"mm1\" -> 0.000048616206   ,  \"mm2\" -> 0.013163310838   ,  \"mm3\" -> 0.016423248374   ,  \"T\" -> 1.900000000000   ,  \"B\" -> 12.000000000000   ,  \"θ\" -> 30.000000000000   ,  \"Reoff\" -> 0.000000000000   ,  \"Imoff\" -> 0.000000000000   ,  \"στ1\" -> 0.000000000000   ,  \"στS\" -> 0.000000000000   ,  \"στN\" -> 0.000000000000    |>   , \n\"IDS0293_210427_RAW_cal__sam_\" ->   <|    \"ζ\" -> 0.009769235649   ,  \"τ1\" -> 0.020538276815   ,  \"τS\" -> 0.013494754544   ,  \"τN\" -> 0.000177075548   ,  \"τC\" -> 0.005872879859   ,  \"κ0\" -> 0.000000013933   ,  \"mm1\" -> 0.000039786676   ,  \"mm2\" -> 0.018120715591   ,  \"mm3\" -> 0.022056047829   ,  \"T\" -> 1.900000000000   ,  \"B\" -> 12.000000000000   ,  \"θ\" -> 30.000000000000   ,  \"Reoff\" -> -172000.000000000000   ,  \"Imoff\" -> 0.000000000000   ,  \"στ1\" -> 0.000000000000   ,  \"στS\" -> 0.000000000000   ,  \"στN\" -> 0.000000000000    |>   , \n\"IDS0294_210427_RAW_cal__ref_\" ->   <|    \"ζ\" -> 0.017975147456   ,  \"τ1\" -> 0.015573317032   ,  \"τS\" -> 0.016697357463   ,  \"τN\" -> 0.000401487663   ,  \"τC\" -> 0.004243374884   ,  \"κ0\" -> 0.000000007622   ,  \"mm1\" -> 0.000060128790   ,  \"mm2\" -> 0.014656172673   ,  \"mm3\" -> 0.022506589842   ,  \"T\" -> 1.130000000000   ,  \"B\" -> 12.000000000000   ,  \"θ\" -> 30.000000000000   ,  \"Reoff\" -> 0.000000000000   ,  \"Imoff\" -> 0.000000000000   ,  \"στ1\" -> 0.000000000000   ,  \"στS\" -> 0.000000000000   ,  \"στN\" -> 0.000000000000    |>   , \n\"IDS0294_210427_RAW_cal__sam_\" ->   <|    \"ζ\" -> 0.010952304636   ,  \"τ1\" -> 0.020329649306   ,  \"τS\" -> 0.020621176960   ,  \"τN\" -> 0.000487558003   ,  \"τC\" -> 0.005477732780   ,  \"κ0\" -> 0.000000008194   ,  \"mm1\" -> 0.000047079068   ,  \"mm2\" -> 0.019035053021   ,  \"mm3\" -> 0.028065174256   ,  \"T\" -> 1.130000000000   ,  \"B\" -> 12.000000000000   ,  \"θ\" -> 30.000000000000   ,  \"Reoff\" -> -250000.000000000000   ,  \"Imoff\" -> 0.000000000000   ,  \"στ1\" -> 0.000000000000   ,  \"στS\" -> 0.000000000000   ,  \"στN\" -> 0.000000000000    |>   , \n\"IDS0295_210427_RAW_cal__ref_\" ->   <|    \"ζ\" -> 0.021360373560   ,  \"τ1\" -> 0.017226807214   ,  \"τS\" -> 0.021136224671   ,  \"τN\" -> 0.000857882935   ,  \"τC\" -> 0.004088468956   ,  \"κ0\" -> 0.000000005432   ,  \"mm1\" -> 0.000072090186   ,  \"mm2\" -> 0.015812919970   ,  \"mm3\" -> 0.027894175974   ,  \"T\" -> 0.830000000000   ,  \"B\" -> 12.000000000000   ,  \"θ\" -> 30.000000000000   ,  \"Reoff\" -> 0.000000000000   ,  \"Imoff\" -> 0.000000000000   ,  \"στ1\" -> 0.000000000000   ,  \"στS\" -> 0.000000000000   ,  \"στN\" -> 0.000000000000    |>   , \n\"IDS0295_210427_RAW_cal__sam_\" ->   <|    \"ζ\" -> 0.014046811833   ,  \"τ1\" -> 0.021205417259   ,  \"τS\" -> 0.025982453768   ,  \"τN\" -> 0.000985536826   ,  \"τC\" -> 0.005692013080   ,  \"κ0\" -> 0.000000005890   ,  \"mm1\" -> 0.000064969808   ,  \"mm2\" -> 0.019619534974   ,  \"mm3\" -> 0.034559730440   ,  \"T\" -> 0.830000000000   ,  \"B\" -> 12.000000000000   ,  \"θ\" -> 30.000000000000   ,  \"Reoff\" -> -401999.999999999999   ,  \"Imoff\" -> 0.000000000000   ,  \"στ1\" -> 0.000000000000   ,  \"στS\" -> 0.000000000000   ,  \"στN\" -> 0.000000000000    |>   , \n\"IDS0296_210427_RAW_cal__ref_\" ->   <|    \"ζ\" -> 0.027756025784   ,  \"τ1\" -> 0.019742757718   ,  \"τS\" -> 0.026611973171   ,  \"τN\" -> 0.001398943183   ,  \"τC\" -> 0.003482574473   ,  \"κ0\" -> 0.000000003907   ,  \"mm1\" -> 0.000083653758   ,  \"mm2\" -> 0.017774350196   ,  \"mm3\" -> 0.034155716307   ,  \"T\" -> 0.620000000000   ,  \"B\" -> 12.000000000000   ,  \"θ\" -> 30.000000000000   ,  \"Reoff\" -> 0.000000000000   ,  \"Imoff\" -> 0.000000000000   ,  \"στ1\" -> 0.000000000000   ,  \"στS\" -> 0.000000000000   ,  \"στN\" -> 0.000000000000    |>   , \n\"IDS0296_210427_RAW_cal__sam_\" ->   <|    \"ζ\" -> 0.017388662959   ,  \"τ1\" -> 0.016835863979   ,  \"τS\" -> 0.033051741689   ,  \"τN\" -> 0.001876583642   ,  \"τC\" -> 0.004718731610   ,  \"κ0\" -> 0.000000004257   ,  \"mm1\" -> 0.000070854167   ,  \"mm2\" -> 0.015532685015   ,  \"mm3\" -> 0.041486738616   ,  \"T\" -> 0.620000000000   ,  \"B\" -> 12.000000000000   ,  \"θ\" -> 30.000000000000   ,  \"Reoff\" -> -602409.638554215430   ,  \"Imoff\" -> 0.000000000000   ,  \"στ1\" -> 0.000000000000   ,  \"στS\" -> 0.000000000000   ,  \"στN\" -> 0.000000000000    |>   , \n\"IDS0297_210427_RAW_cal__ref_\" ->   <|    \"ζ\" -> 0.034775017342   ,  \"τ1\" -> 0.018923965005   ,  \"τS\" -> 0.030086686370   ,  \"τN\" -> 0.002286572055   ,  \"τC\" -> 0.002714831651   ,  \"κ0\" -> 0.000000003294   ,  \"mm1\" -> 0.000084124720   ,  \"mm2\" -> 0.016628755460   ,  \"mm3\" -> 0.038424955523   ,  \"T\" -> 0.530000000000   ,  \"B\" -> 12.000000000000   ,  \"θ\" -> 30.000000000000   ,  \"Reoff\" -> 0.000000000000   ,  \"Imoff\" -> 0.000000000000   ,  \"στ1\" -> 0.000000000000   ,  \"στS\" -> 0.000000000000   ,  \"στN\" -> 0.000000000000    |>   , \n\"IDS0297_210427_RAW_cal__sam_\" ->   <|    \"ζ\" -> 0.020542184284   ,  \"τ1\" -> 0.020760439172   ,  \"τS\" -> 0.037341907366   ,  \"τN\" -> 0.003219016214   ,  \"τC\" -> 0.004292471555   ,  \"κ0\" -> 0.000000003557   ,  \"mm1\" -> 0.000077795275   ,  \"mm2\" -> 0.018267084885   ,  \"mm3\" -> 0.048102164115   ,  \"T\" -> 0.530000000000   ,  \"B\" -> 12.000000000000   ,  \"θ\" -> 30.000000000000   ,  \"Reoff\" -> -602409.638554215430   ,  \"Imoff\" -> 0.000000000000   ,  \"στ1\" -> 0.000000000000   ,  \"στS\" -> 0.000000000000   ,  \"στN\" -> 0.000000000000    |>   , \n\"IDS0298_210427_RAW_cal__ref_\" ->   <|    \"ζ\" -> 0.046440102993   ,  \"τ1\" -> 0.018907201785   ,  \"τS\" -> 0.034021724611   ,  \"τN\" -> 0.004470088018   ,  \"τC\" -> 0.002281608431   ,  \"κ0\" -> 0.000000002638   ,  \"mm1\" -> 0.000095393981   ,  \"mm2\" -> 0.015614445786   ,  \"mm3\" -> 0.045758346821   ,  \"T\" -> 0.430000000000   ,  \"B\" -> 12.000000000000   ,  \"θ\" -> 30.000000000000   ,  \"Reoff\" -> -3126506.024096369740   ,  \"Imoff\" -> 0.000000000000   ,  \"στ1\" -> 0.013462619776   ,  \"στS\" -> 0.001228313505   ,  \"στN\" -> 0.000000000000    |>   , \n\"IDS0298_210427_RAW_cal__sam_\" ->   <|    \"ζ\" -> 0.028504600675   ,  \"τ1\" -> 0.017787596977   ,  \"τS\" -> 0.043231501144   ,  \"τN\" -> 0.005920795525   ,  \"τC\" -> 0.002978583592   ,  \"κ0\" -> 0.000000002855   ,  \"mm1\" -> 0.000077491236   ,  \"mm2\" -> 0.014973532625   ,  \"mm3\" -> 0.056268519966   ,  \"T\" -> 0.430000000000   ,  \"B\" -> 12.000000000000   ,  \"θ\" -> 30.000000000000   ,  \"Reoff\" -> -2300000.000000000000   ,  \"Imoff\" -> 0.000000000000   ,  \"στ1\" -> 0.000000000000   ,  \"στS\" -> 0.000000000000   ,  \"στN\" -> 0.000000000000    |>   , \n\"IDS0299_210427_RAW_cal__ref_\" ->   <|    \"ζ\" -> 0.060451978173   ,  \"τ1\" -> 0.020932044867   ,  \"τS\" -> 0.038339527687   ,  \"τN\" -> 0.009019484504   ,  \"τC\" -> 0.001991911381   ,  \"κ0\" -> 0.000000002121   ,  \"mm1\" -> 0.000108517518   ,  \"mm2\" -> 0.015468645240   ,  \"mm3\" -> 0.057568751652   ,  \"T\" -> 0.360000000000   ,  \"B\" -> 12.000000000000   ,  \"θ\" -> 30.000000000000   ,  \"Reoff\" -> -4033132.530120491980   ,  \"Imoff\" -> 0.000000000000   ,  \"στ1\" -> 0.008893690340   ,  \"στS\" -> 0.001445462224   ,  \"στN\" -> 0.000000000000    |>   , \n\"IDS0299_210427_RAW_cal__sam_\" ->   <|    \"ζ\" -> 0.036443500348   ,  \"τ1\" -> 0.020154057220   ,  \"τS\" -> 0.048932682096   ,  \"τN\" -> 0.011280238135   ,  \"τC\" -> 0.002753749788   ,  \"κ0\" -> 0.000000002299   ,  \"mm1\" -> 0.000091994249   ,  \"mm2\" -> 0.015410264614   ,  \"mm3\" -> 0.069812837955   ,  \"T\" -> 0.360000000000   ,  \"B\" -> 12.000000000000   ,  \"θ\" -> 30.000000000000   ,  \"Reoff\" -> -2590361.445783123380   ,  \"Imoff\" -> 0.000000000000   ,  \"στ1\" -> 0.000000000000   ,  \"στS\" -> 0.000000000000   ,  \"στN\" -> 0.000000000000    |>   , \n\"IDS0300_210427_RAW_cal__ref_\" ->   <|    \"ζ\" -> 0.339239140566   ,  \"τ1\" -> 0.049004480747   ,  \"τS\" -> 0.154731734875   ,  \"τN\" -> 0.405076937535   ,  \"τC\" -> 0.001214632941   ,  \"κ0\" -> 0.000000000422   ,  \"mm1\" -> 0.000306310339   ,  \"mm2\" -> 0.012966272526   ,  \"mm3\" -> 0.786664216144   ,  \"T\" -> 0.140000000000   ,  \"B\" -> 12.000000000000   ,  \"θ\" -> 30.000000000000   ,  \"Reoff\" -> -103762048.192771077000   ,  \"Imoff\" -> 0.000000000000   ,  \"στ1\" -> 0.015510670555   ,  \"στS\" -> 0.015380063166   ,  \"στN\" -> 0.000000000000    |>   , \n\"IDS0300_210427_RAW_cal__sam_\" ->   <|    \"ζ\" -> 0.180438460866   ,  \"τ1\" -> 0.048255220427   ,  \"τS\" -> 0.195496614309   ,  \"τN\" -> 0.254134303670   ,  \"τC\" -> 0.001384159230   ,  \"κ0\" -> 0.000000000598   ,  \"mm1\" -> 0.000210501936   ,  \"mm2\" -> 0.019979803647   ,  \"mm3\" -> 0.560210702851   ,  \"T\" -> 0.140000000000   ,  \"B\" -> 12.000000000000   ,  \"θ\" -> 30.000000000000   ,  \"Reoff\" -> -29759036.144578307900   ,  \"Imoff\" -> 0.000000000000   ,  \"στ1\" -> 0.000000000000   ,  \"στS\" -> 0.000000000000   ,  \"στN\" -> 0.000000000000    |>   , \n\"IDS0301_210831_RAW_cal__ref_\" ->   <|    \"ζ\" -> 0.083102815664   ,  \"τ1\" -> 0.023587336655   ,  \"τS\" -> 0.043380203208   ,  \"τN\" -> 0.014582503470   ,  \"τC\" -> 0.001563516475   ,  \"κ0\" -> 0.000000001737   ,  \"mm1\" -> 0.000116373060   ,  \"mm2\" -> 0.015882403600   ,  \"mm3\" -> 0.071931647277   ,  \"T\" -> 0.300000000000   ,  \"B\" -> 12.000000000000   ,  \"θ\" -> 30.000000000000   ,  \"Reoff\" -> -7370481.927710846070   ,  
